vi "AutoCorrelation Matrix.vi"   [LabVIEW 2020, in "NI_AAL_SigProc.lvlib"]
doc: "Computes the autocorrelation matrix of the input sequence <B>X</B>. Wire data to the <B>X</B> input to determine the polymorphic instance to use or manually select the instance."
uses:
  <vilib>/Analysis/NI_AAL_SigProc.lvlib
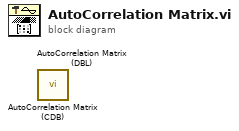
[diagram p0: block diagram]
diagram:
  n1 = call <vilib>:"AutoCorrelation Matrix (CDB).vi"() -> ()  [unwired: 10 in, 2 out]
  n2 = call <vilib>:"AutoCorrelation Matrix (DBL).vi"() -> ()  [unwired: 10 in, 2 out]
